vi "Template Files Path.vi"() -> (1 "default template path":path, 2 "template lib path":path, 3 "xydata ctl path":path)   [LabVIEW 2021, in "NI Measurement V2 Client Generator Runtime.lvlib"]
uses:
  NI Measurement V2 Client Generator Runtime.lvlib
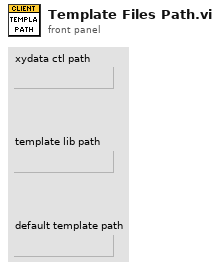
[diagram p1: front panel]
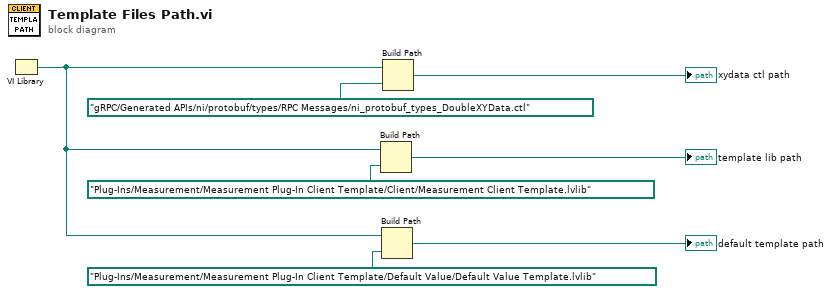
[diagram p0: block diagram]
diagram:
  n1 = VI Library() -> (path=w1:path)
  n2 = Build Path(base path=w1, name or relative path=path "Plug-Ins/Measurement/Measurement Plug-In Client Template/Client/Measurement Client Template.lvlib") -> (appended path=→"template lib path":path)
  n3 = Build Path(base path=w1, name or relative path=path "Plug-Ins/Measurement/Measurement Plug-In Client Template/Default Value/Default Value Template.lvlib") -> (appended path=→"default template path":path)
  n4 = Build Path(base path=w1, name or relative path=path "gRPC/Generated APIs/ni/protobuf/types/RPC Messages/ni_protobuf_types_DoubleXYData.ctl") -> (appended path=→"xydata ctl path":path)
